vi "RW-BC.vi"() -> ()   [LabVIEW 2020]
uses:
  <vilib>/addons/database/_DB Variant To Data/Database Variant To Data.xnode
  <vilib>/addons/database/NI_Database_API.lvlib
panel:
  in  "Boolean":bool=TRUE
  out "Currency from DB":dbl
  out "Boolean from DB":bool
  in  "Currency":dbl
  in  "error in (no error)":errorcluster
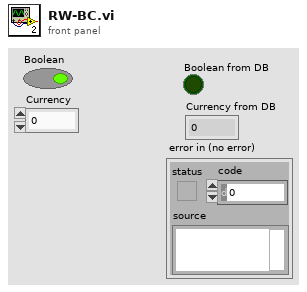
[diagram p1: front panel]
types:
  T1 = typedef "NI_Database_API.lvlib/Conn ObjectReference.ctl" = refnum<k1>
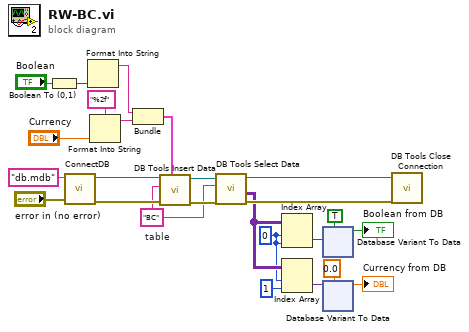
[diagram p0: block diagram]
diagram:
  w8 = 0 ("index (row)")
  w12 = "BC"  # table
  n1 = Boolean To (0,1)(Boolean="Boolean") -> (0, 1=w21:i16)
  n2 = call "ConnectDB.vi"("error in (no error)"="error in (no error)", "Filename"="db.mdb") -> ("error out"=w22:errorcluster, "DB Conn"=w23:T1)  [unwired: 8 in]
  n3 = Format Into String(w21) -> (resulting string=w19:string)  [unwired: 3 in, 1 out]
  n4 = Format Into String(format string="%2f", "Currency") -> (resulting string=w16:string)  [unwired: 2 in, 1 out]
  n5 = Bundle(w19, w16) -> (w15:cluster{string, string})  [unwired: 1 in]
  n6 = call <vilib>:"DB Tools Insert Data.vi"("data"=w15, "error in (no error)"=w22, "table"=w12, "connection reference"=w23) -> ("error out"=w13:errorcluster, "connection reference out"=w14:T1)  [unwired: 6 in]
  n7 = call <vilib>:"DB Tools Select Data.vi"("error in (no error)"=w13, "table"=w12, "connection reference"=w14) -> ("error out"=w10:errorcluster, "data"=w9:variant[][], "connection reference out"=w11:T1)  [unwired: 3 in]
  n8 = Index Array(array=w9, index (row)=w8, index (col)=w8) -> (element=w6:variant)
  n9 = Index Array(array=w9, index (row)=w8, index (col)=1 ("disabled index (col)")) -> (element=w5:variant)
  n10 = xnode "Database Variant To Data"("database variant"=w6, "type"=TRUE) -> ("data"=→"Boolean from DB":bool)  [unwired: 1 in, 1 out]
  n11 = xnode "Database Variant To Data"("database variant"=w5, "type"=0.0) -> ("data"=→"Currency from DB":dbl)  [unwired: 1 in, 1 out]
  n12 = call <vilib>:"DB Tools Close Connection.vi"("error in (no error)"=w10, "connection reference"=w11) -> ()  [unwired: 5 in, 1 out]
